vi "dfd_Group Delay_Initial Value.vi"(8 "error in (no error)":errorcluster, 10 "initial guess":cluster{"iteration times":i32, "seed":dbl}={"iteration times"=5, "seed"=1.0}, 11 "Design Info":T2={"p"=2, "freq grid"=[], "d"=[], "weight"=[], "Order"=0, "radius"=0.0}) -> (0 "error out":errorcluster, 2 "Coefficients":T1(array[cluster]), 3 "Design Info (dup)":T2={"p"=2, "freq grid"=[], "d"=[], "weight"=[], "Order"=0, "radius"=0.0})   [LabVIEW 2017, in "NI_DigFilter_Design.lvlib"]
uses:
  <vilib>/addons/Digital Filter Design/NI_DigFilter_Design.lvlib
  <vilib>/addons/Digital Filter Design/_GroupDelay.llb/dfd_Group Delay_Design Info.ctl
  <vilib>/addons/Digital Filter Design/_Misc.llb/dfd_Error Handlers (Single).vi
  <vilib>/addons/Digital Filter Design/NI_DigFilterLicensed.lvlib
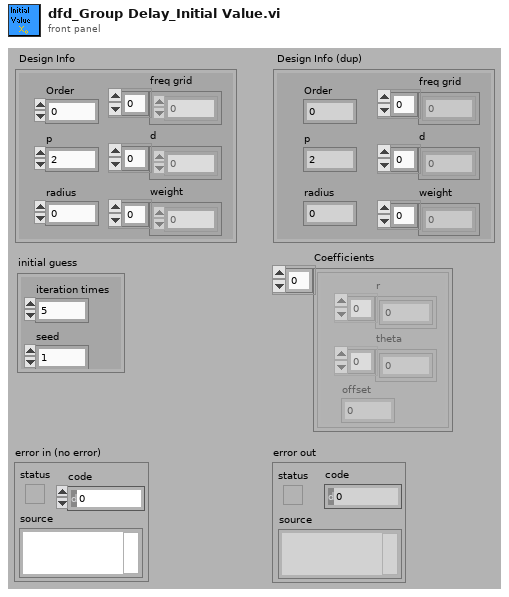
[diagram p1: front panel]
types:
  T1 = cluster{"r":dbl[], "theta":dbl[], "offset":dbl}[]
  T2 = typedef "dfd_Group Delay_Design Info.ctl" = cluster{"p":i32, "freq grid":dbl[], "d":dbl[], "weight":dbl[], "Order":i32, "radius":dbl}
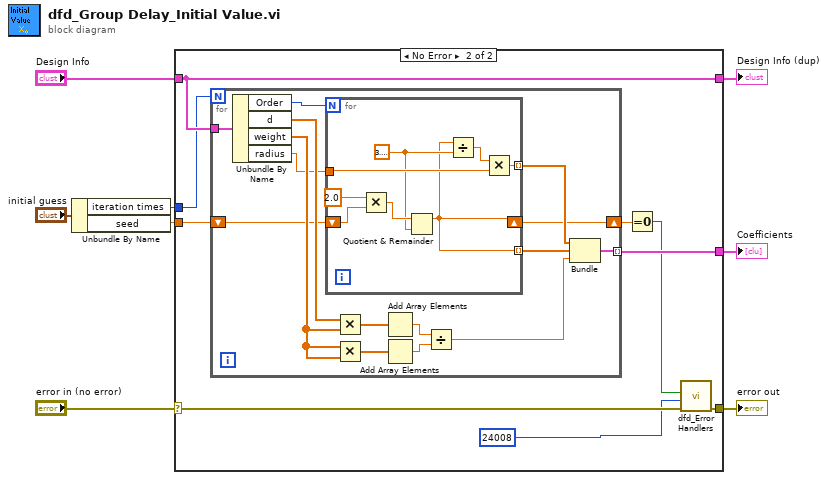
[diagram p0: block diagram]
diagram:
  n1 = Unbundle By Name("initial guess") -> ("iteration times"=w3:i32, "seed"=w2:dbl)
  n2 = case shown="No Error" "error in (no error)" {
    selector: "error in (no error)" -> [w9 w13]
    tunnel: "Design Info" -> [w10 w18]
    tunnel: [_ w19] -> w1
    tunnel: [w9 w14] -> w6
    tunnel: [w10 w18] -> w5
    tunnel: w3 -> [_ w16]
    tunnel: w2 -> [_ w17]
    frame Error {
    }
    frame No Error {
      n3 = for {
        N: w16 -> [_]
        tunnel: w18 -> [w24]
        tunnel: [w23] -> w19 mode=indexing
        shift-right: [w21] -> w15
        shift-left: w17 -> [w22]
        n4 = Unbundle By Name(w24) -> ("Order"=w34:i32, "d"=w31:dbl[], "weight"=w30:dbl[], "radius"=w20:dbl)
        n5 = for {
          N: w34 -> [_]
          tunnel: [w37] -> w33 mode=indexing
          tunnel: [w35] -> w32 mode=indexing
          tunnel: w20 -> [w38]
          shift-right: [w35] -> w21
          shift-left: w22 -> [w42]
          w36 = 3.141592653589793
          n6 = Multiply(x=2.0, y=w42) -> (x*y=w40:dbl)
          n7 = Quotient & Remainder(x=w40, y=w36) -> (x-y*floor(x/y)=w35:dbl)  [unwired: 1 out]
          n8 = Divide(x=w35, y=w36) -> (x/y=w39:dbl)
          n9 = Multiply(x=w39, y=w38) -> (x*y=w37:dbl)
        }
        n10 = Multiply(x=w31, y=w30) -> (x*y=w29:dbl[])
        n11 = Multiply(x=w30, y=w30) -> (x*y=w28:dbl[])
        n12 = Add Array Elements(numeric array=w29) -> (sum=w27:dbl)
        n13 = Add Array Elements(numeric array=w28) -> (sum=w26:dbl)
        n14 = Divide(x=w27, y=w26) -> (x/y=w25:dbl)
        n15 = Bundle(w33, w32, w25) -> (w23:cluster{dbl[], dbl[], dbl})  [unwired: 1 out]
      }
      n16 = Equal To 0?(x=w15) -> (x = 0?=w12:bool)
      n17 = call-poly <vilib>:"dfd_Error Handlers.vi"("error in (no error)"=w13, "error code"=24008 ("WRN_INI_GUESS_SEED"), "condition failed?"=w12) -> ("error out"=w14:errorcluster)  [unwired: 8 out]
    }
  }
  "Design Info (dup)" <- w5
  "error out" <- w6
  "Coefficients" <- w1
